vi "moveNode.vi"(8 "error in (no error)":errorcluster, 9 "Direction":T1, 10 "Node Path":string, 11 "xceRootNode in":refnum<class "xceRootNode.lvclass">) -> (0 "error out":errorcluster, 3 "xceRootNode out":refnum<class "xceRootNode.lvclass">)   [LabVIEW 2013, in "xceRootNode.lvclass"]
doc: "Moves a node either up or down with relationship to the nodes with the same supernode."
uses:
  xceRootNode.lvclass
  moveDirection.ctl
  xceDataNode/xceDataNode.lvclass
  xceRootNode.lvclass/xceRootNode.ctl
  xceNode/xceNode.lvclass
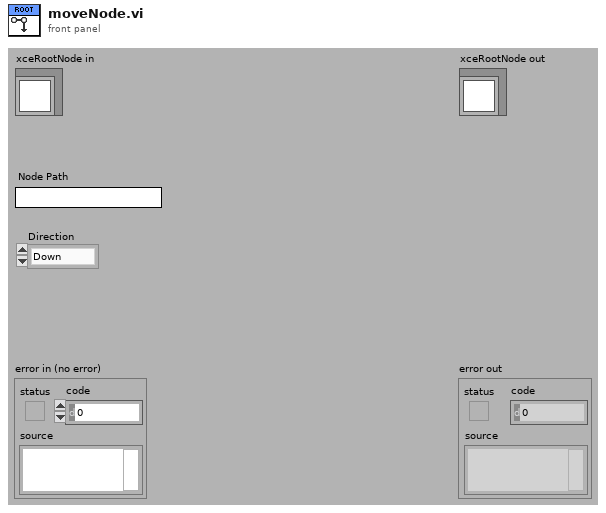
[diagram p1: front panel]
types:
  T1 = typedef "xceRootNode.lvclass/moveDirection.ctl" = enum16{"Down", "Up"}
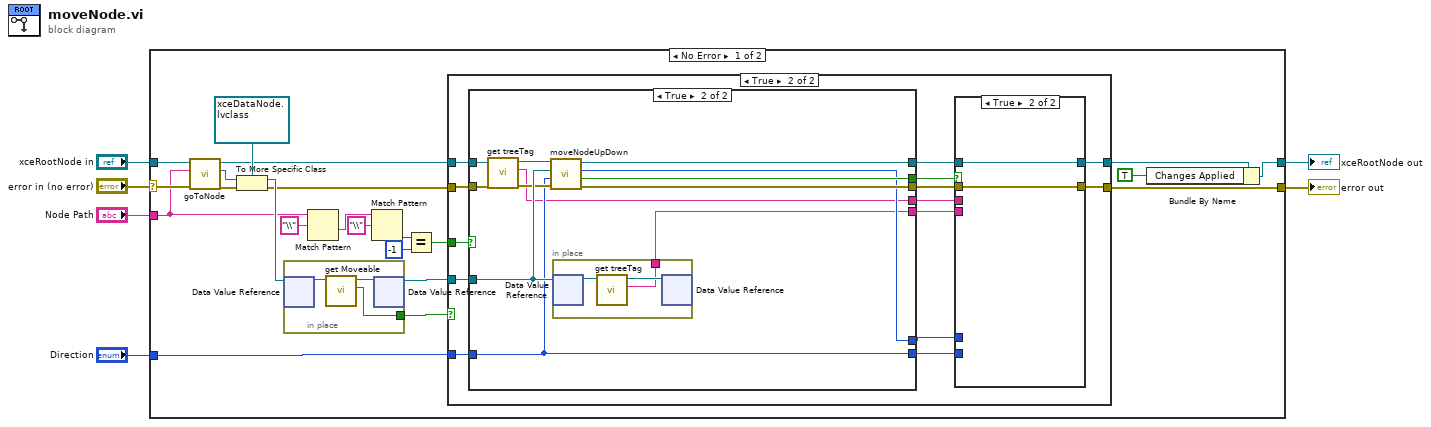
[diagram p0: block diagram]
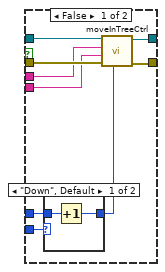
[diagram p3: hidden frame]
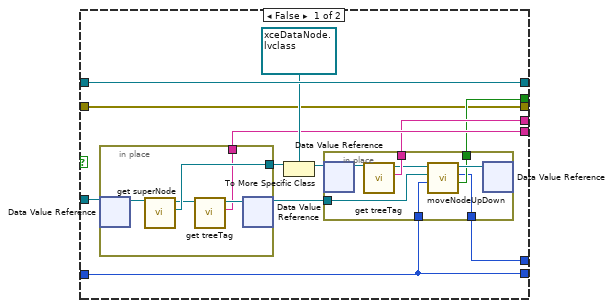
[diagram p5: hidden frame]
diagram:
  n1 = case shown="No Error" "error in (no error)" {
    selector: "error in (no error)" -> [w27 w103]
    tunnel: [w18 w103] -> w5
    tunnel: [w7 w102] -> w3
    tunnel: "xceRootNode in" -> [w28 w102]
    tunnel: "Node Path" -> [w17 _]
    tunnel: "Direction" -> [w10 _]
    frame No Error {
      n2 = call "goToNode.vi"("error in (no error)"=w27, "Node Path"=w17, "xceNode in"=w28) -> ("error out"=w25:errorcluster, "goToNode* out"=w26:refnum<data-value>, "xceNode out"=w22:refnum<class "xceRootNode.lvclass">)  [unwired: 6 in]
      n3 = To More Specific Class(target class=refnum<data-value> refnum ("data value reference"), reference=w26, error in=w25) -> (specific class reference=w23:refnum<data-value>, error out=w19:errorcluster)
      n4 = in-place {
        in-place-border: [w99] -> w21
        n5 = in-place-dvr #1(w23) -> (w100:refnum<class "xceDataNode.lvclass">)  [unwired: 1 out]
        n6 = call "get Moveable.vi"("xceDataNode in"=w100) -> ("Moveable"=w99:bool, "xceDataNode out"=w101:refnum<class "xceDataNode.lvclass">)  [unwired: 8 in, 1 out]
        n7 = in-place-dvr #1(w101) -> (w20:refnum<data-value>)  [unwired: 1 out]
      }
      n8 = Match Pattern(string=w17, regular expression="\\") -> (after substring=w15:string)  [unwired: 1 in, 3 out]
      n9 = Match Pattern(string=w15, regular expression="\\") -> (offset past match=w13:i32)  [unwired: 1 in, 3 out]
      n10 = Equal?(x=w13, y=-1) -> (x = y?=w11:bool)
      n11 = case shown="True" w21 {
        tunnel: w22 -> [w30 w43]
        tunnel: w20 -> [_ w41]
        tunnel: [w30 w37] -> w9
        tunnel: w19 -> [w29 w42]
        tunnel: [w29 w35] -> w18
        tunnel: w11 -> [_ w44]
        tunnel: w10 -> [_ w40]
        frame False {
        }
        frame True {
          n12 = case shown="True" w44 {
            tunnel: w43 -> [w70 w91]
            tunnel: w42 -> [w59 w89]
            tunnel: w41 -> [w69 w92]
            tunnel: w40 -> [w60 w86]
            tunnel: [w70 w95] -> w38
            tunnel: [w62 w94] -> w39
            tunnel: [w59 w93] -> w36
            tunnel: [w61 w87] -> w34
            tunnel: [w60 w86] -> w33
            tunnel: [w64 w85] -> w32
            tunnel: [w66 w84] -> w31
            frame False {
              n13 = in-place {
                in-place-border: [w82] -> w67
                in-place-border: [w79] -> w66
                n14 = in-place-dvr #2(w69) -> (w83:refnum<class "xceDataNode.lvclass">)  [unwired: 1 out]
                n15 = call "get superNode.vi"("xceNode in"=w83) -> ("superNode*"=w82:refnum<data-value>, "xceNode out"=w81:refnum<class "xceDataNode.lvclass">)  [unwired: 8 in, 1 out]
                n16 = call "get treeTag.vi"("xceNode in"=w81) -> ("treeTag"=w79:string, "xceNode out"=w80:refnum<class "xceDataNode.lvclass">)  [unwired: 8 in, 1 out]
                n17 = in-place-dvr #2(w80) -> (w63:refnum<data-value>)  [unwired: 1 out]
              }
              n18 = To More Specific Class(target class=refnum<data-value> refnum ("data value reference"), reference=w67) -> (specific class reference=w65:refnum<data-value>)  [unwired: 1 in, 1 out]
              n19 = in-place {
                in-place-border: [w77] -> w64
                in-place-border: w63 -> [w74]
                in-place-border: w60 -> [w73]
                in-place-border: [w72] -> w62
                in-place-border: [w71] -> w61
                n20 = in-place-dvr #3(w65) -> (w78:refnum<class "xceDataNode.lvclass">)  [unwired: 1 out]
                n21 = call "get treeTag.vi"("xceNode in"=w78) -> ("treeTag"=w77:string, "xceNode out"=w76:refnum<class "xceDataNode.lvclass">)  [unwired: 8 in, 1 out]
                n22 = call "moveNodeUpDown.vi"("Direction"=w73, "subNode* in"=w74, "superNode in"=w76) -> ("No Change"=w72:bool, "new Index"=w71:i32, "superNode out"=w75:refnum<class "xceDataNode.lvclass">)  [unwired: 5 in, 1 out]
                n23 = in-place-dvr #3(w75) -> ()  [unwired: 2 out]
              }
            }
            frame True {
              n24 = call "get treeTag.vi"("error in (no error)"=w89, "xceNode in"=w91) -> ("error out"=w88:errorcluster, "treeTag"=w85:string, "xceNode out"=w90:refnum<class "xceRootNode.lvclass">)  [unwired: 7 in]
              n25 = call "moveNodeUpDown.vi"("error in (no error)"=w88, "Direction"=w86, "subNode* in"=w92, "superNode in"=w90) -> ("error out"=w93:errorcluster, "No Change"=w94:bool, "new Index"=w87:i32, "superNode out"=w95:refnum<class "xceRootNode.lvclass">)  [unwired: 4 in]
              n26 = in-place {
                in-place-border: [w96] -> w84
                n27 = in-place-dvr #4(w92) -> (w98:refnum<class "xceDataNode.lvclass">)  [unwired: 1 out]
                n28 = call "get treeTag.vi"("xceNode in"=w98) -> ("treeTag"=w96:string, "xceNode out"=w97:refnum<class "xceDataNode.lvclass">)  [unwired: 8 in, 1 out]
                n29 = in-place-dvr #4(w97) -> ()  [unwired: 2 out]
              }
            }
          }
          n30 = case shown="True" w39 {
            tunnel: w38 -> [w53 w58]
            tunnel: [w46 w58] -> w37
            tunnel: w36 -> [w52 w57]
            tunnel: [w45 w57] -> w35
            tunnel: w34 -> [w50 _]
            tunnel: w33 -> [w51 _]
            tunnel: w32 -> [w48 _]
            tunnel: w31 -> [w47 _]
            frame False {
              n31 = case shown="\"Down\", Default" w51 {
                tunnel: w50 -> [w54 w56]
                tunnel: [w55 w56] -> w49
                frame "Down", Default {
                  n32 = Increment(x=w54) -> (x+1=w55:i32)
                }
                frame "Up" {
                }
              }
              n33 = call "moveInTreeCtrl.vi"("Position"=w49, "error in (no error)"=w52, "subNode tag"=w47, "superNode tag"=w48, "xceRootNode in"=w53) -> ("error out"=w45:errorcluster, "xceRootNode out"=w46:refnum<class "xceRootNode.lvclass">)  [unwired: 5 in]
            }
            frame True {
            }
          }
        }
      }
      n34 = Bundle By Name(cluster=w9, "Changes Applied"=TRUE) -> (w7:refnum<class "xceRootNode.lvclass">)
    }
    frame Error {
    }
  }
  "error out" <- w5
  "xceRootNode out" <- w3
